vi "DAQmx.44xx.Get DAQ Type from Task.vi"(8 "error in (no error)":errorcluster, 11 "Task in":refnum<k21>) -> (0 "error out":errorcluster, 1 "DevIsSimulated":bool, 2 "DAQ Type":T1, 3 "Task out":refnum<k21>, 5 "Device":tag)   [LabVIEW 2019, in "DAQmx.lvclass"]
uses:
  DAQmx.lvclass
  typedefs/DAQ.Config.Device Type--enum.ctl
  <resource>/objmgr/daqmx.rc
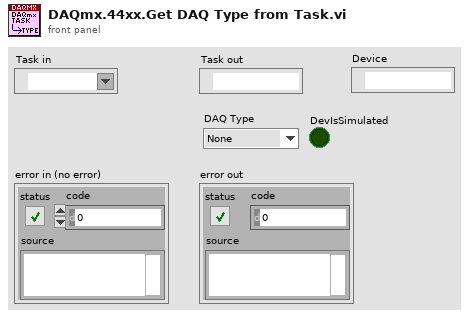
[diagram p1: front panel]
types:
  T1 = typedef "DAQmx.lvclass/DAQ.Config.Device Type--enum.ctl" = enum16{"None", "USB-4431", "PXI-446x"}
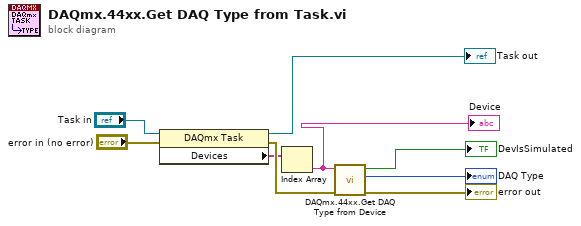
[diagram p0: block diagram]
diagram:
  n1 = property class="DAQmx Task"(reference="Task in", error in="error in (no error)") -> (reference out=→"Task out":refnum<k21>, error out=w8:errorcluster, "Devices"=w3:tag[])
  n2 = Index Array(array=w3) -> (element=w1:tag)  [unwired: 1 in]
  "Device" <- w1
  n3 = call "DAQmx.44xx.Get DAQ Type from Device.vi"("error in (no error)"=w8, "DAQmx Device Name"=w1) -> ("error out"=→"error out":errorcluster, "DAQ Type"=→"DAQ Type":T1, "DevIsSimulated"=→"DevIsSimulated":bool)  [unwired: 7 in]
